vi "From 2D Path Tree Data.vi"(11 "Tree Data":refnum<class "Tree Data.lvclass">) -> (2 "2D Path":path[][](array[path]))   [LabVIEW 2020, in "NI_VIAnCFGDataStructure.lvlib" / "2D Path.lvclass"]
doc: "Extract a 2D Path value from Tree Data type."
uses:
  <vilib>/addons/analyzer/VIAnCFGDataStructure/Data Types/2D Path/2D Path.lvclass
  <vilib>/addons/analyzer/VIAnCFGDataStructure/Tree Data/Tree Data.lvclass
  <vilib>/addons/analyzer/VIAnCFGDataStructure/Data Types/2D Path/2D Path.lvclass/2D Path.ctl
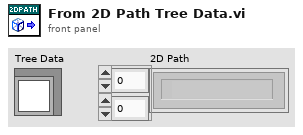
[diagram p1: front panel]
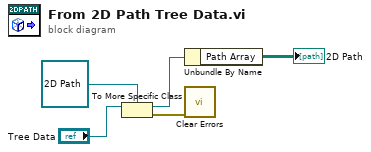
[diagram p0: block diagram]
diagram:
  n1 = To More Specific Class(target class=refnum<class "2D Path.lvclass"> refnum ("Tree API.lvlib:2D Path.lvclass"), reference="Tree Data") -> (specific class reference=w3:refnum<class "2D Path.lvclass">, error out=w2:errorcluster)  [unwired: 1 in]
  n2 = Unbundle By Name(w3) -> ("Path Array"=→"2D Path":path[][])
  n3 = call <vilib>:"Clear Errors.vi"("error in (no error)"=w2) -> ()  [unwired: 5 in, 2 out]
